vi "Error Query.vi"(8 "error in (no error)":errorcluster, 10 "Instrument Message":string[](array[string]), 11 "VISA resource name":refnum<visa-resource-name>) -> (0 "error out":errorcluster, 1 "Error Message":string, 2 "Error Code":i32[](array[numeric]), 3 "VISA resource out":refnum<visa-resource-name>)   [LabVIEW 2011, in "Hokuyo URG Series.lvlib"]
doc: "This VI checks the echo and status byte returned by URG commands and returns an error if one has occured. This VI is only called within the query instrument VI. The error codes used by this driver are documented on the Block Diagram of this VI."
uses:
  Hokuyo URG Series.lvlib
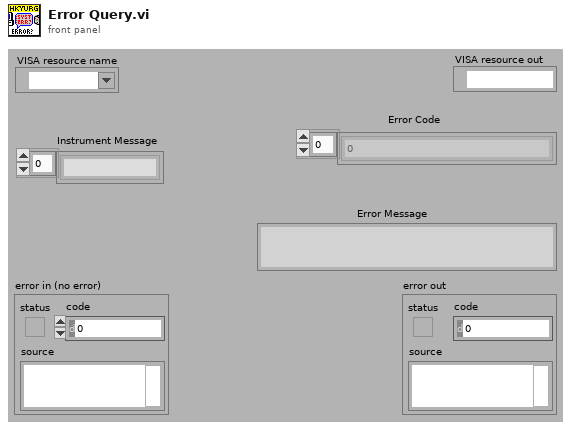
[diagram p1: front panel]
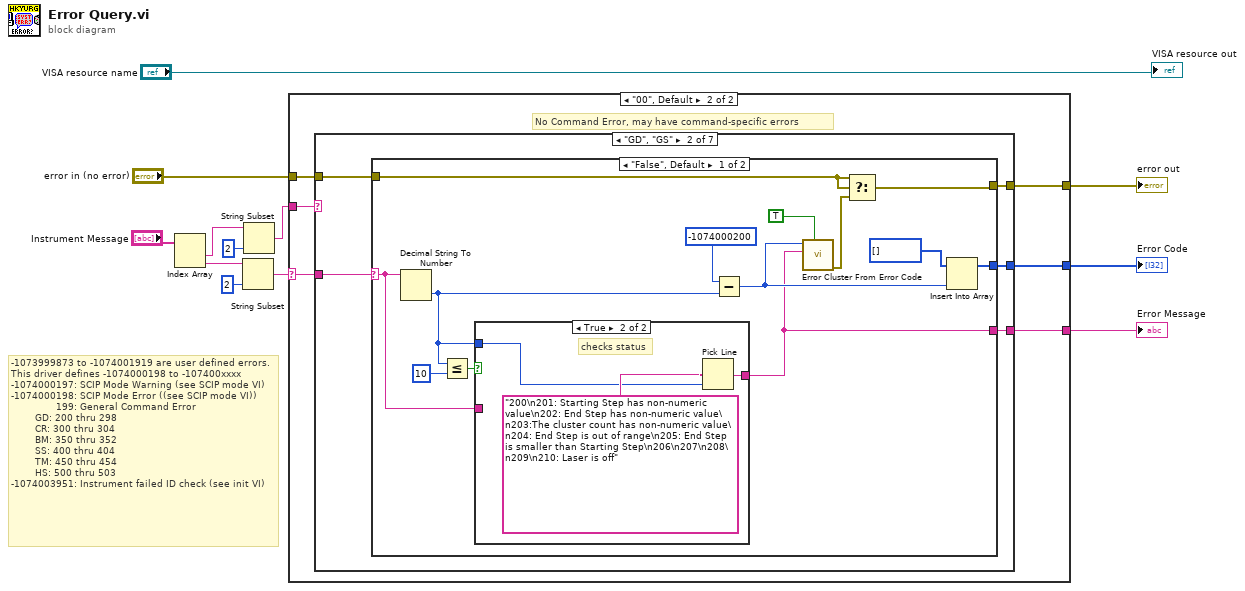
[diagram p0: block diagram]
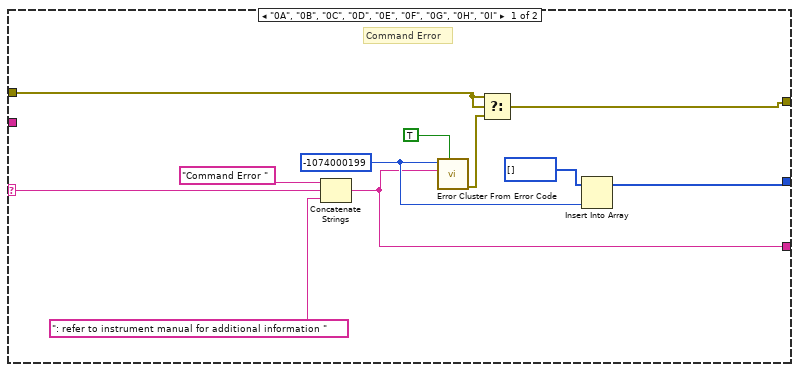
[diagram p2: hidden frame]
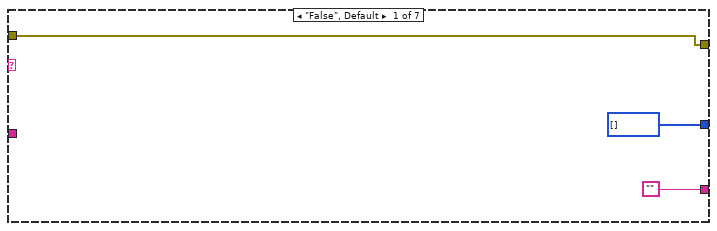
[diagram p3: hidden frame]
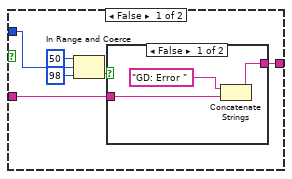
[diagram p4: hidden frame]
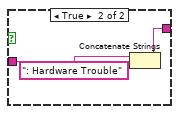
[diagram p5: hidden frame]
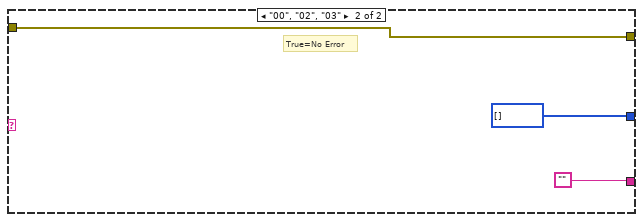
[diagram p6: hidden frame]
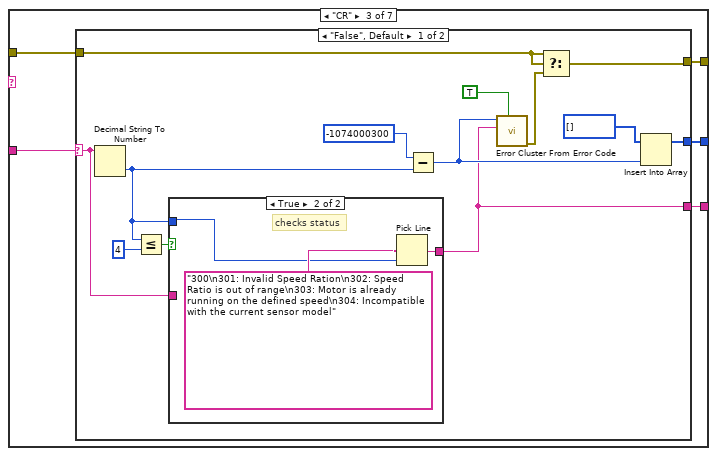
[diagram p7: hidden frame]
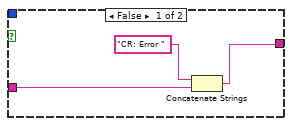
[diagram p8: hidden frame]
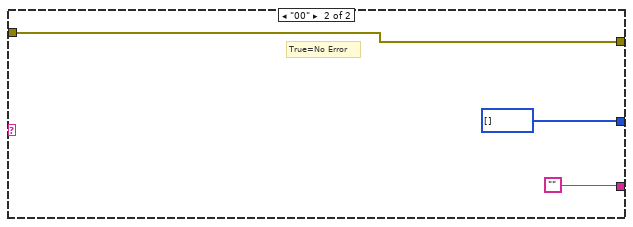
[diagram p9: hidden frame]
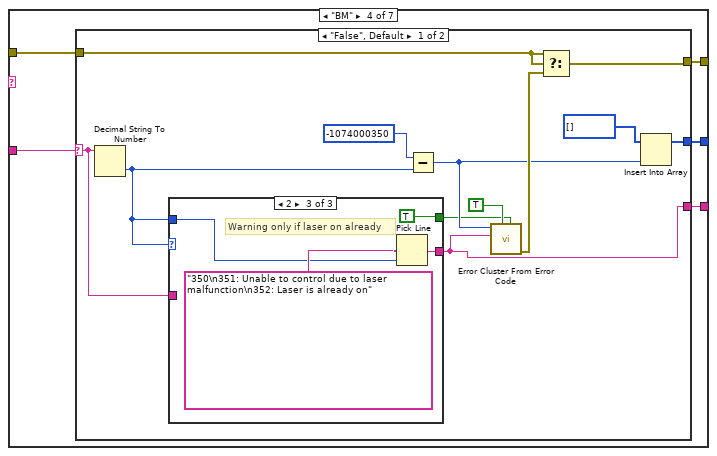
[diagram p10: hidden frame]
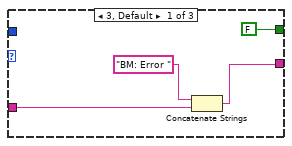
[diagram p11: hidden frame]
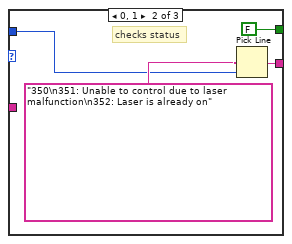
[diagram p12: hidden frame]
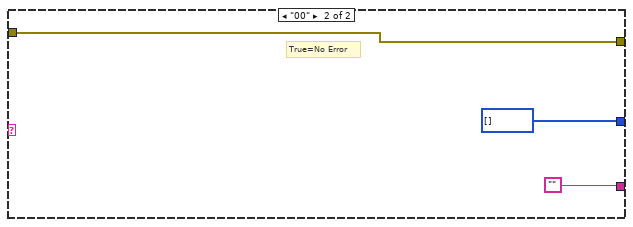
[diagram p13: hidden frame]
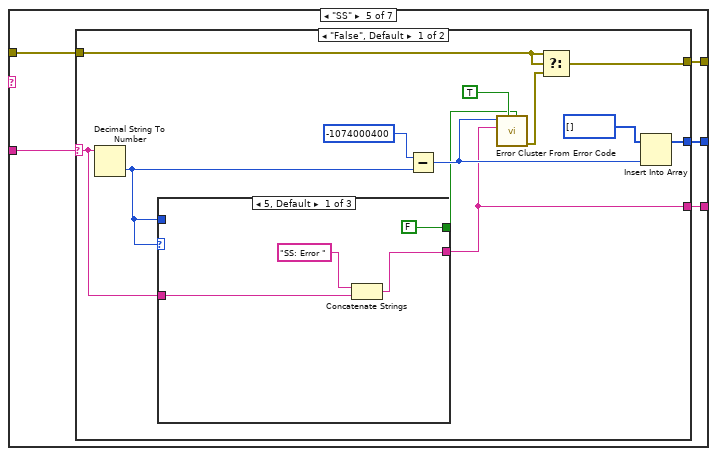
[diagram p14: hidden frame]
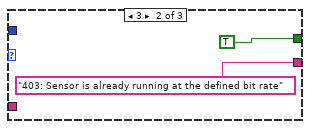
[diagram p15: hidden frame]
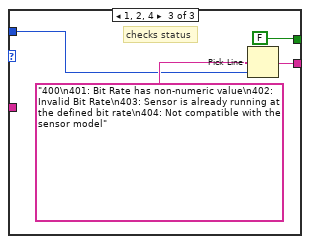
[diagram p16: hidden frame]
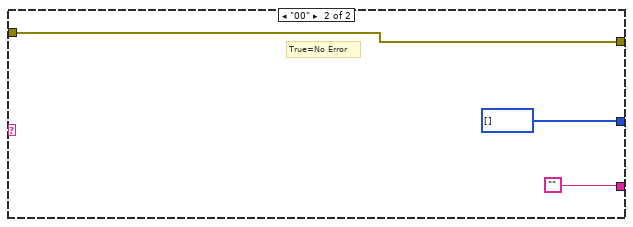
[diagram p17: hidden frame]
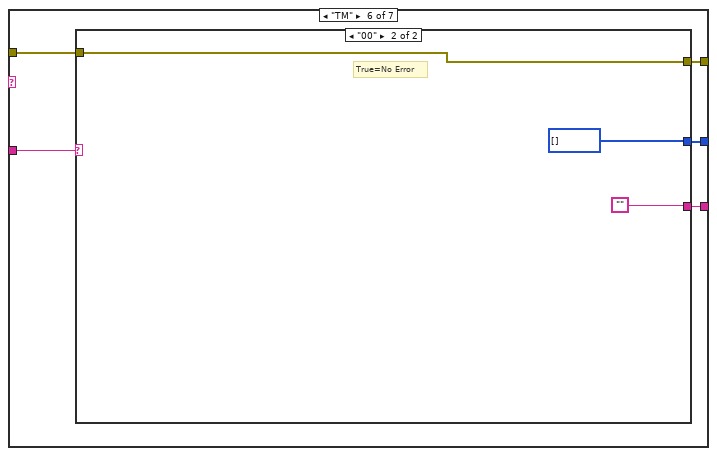
[diagram p18: hidden frame]
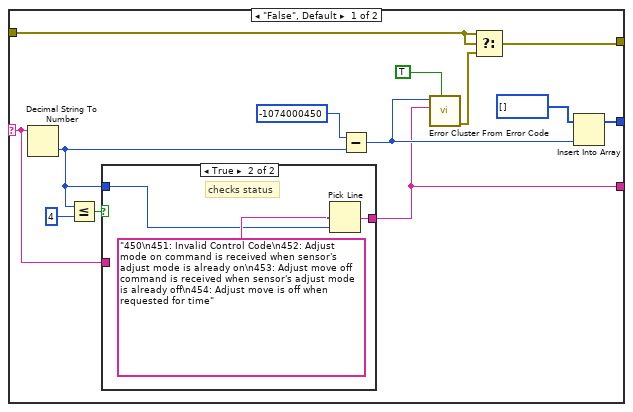
[diagram p19: hidden frame]
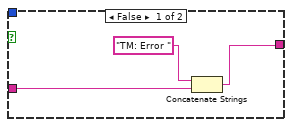
[diagram p20: hidden frame]
diagram:
  # "-1073999873 to -1074001919 are user defined errors.  This driver defines -1074000198 to -107400xxxx\n-1074000197: SCIP Mode Warning (see SCIP mode VI)\n-1074000198: SCIP Mode Error ((see SCIP mode VI))\n               199: General Command Error\n        GD: 200 thru 298\n        CR: 300 thru 304\n        BM: 350 thru 352\n        SS: 400 thru 404\n        TM: 450 thru 454\n        HS: 500 thru 503\n-1074003951: Instrument failed ID check (see init VI)"
  n1 = Index Array(array="Instrument Message") -> (element #1=w3:string, element #2=w4:string)  [unwired: 2 in]
  n2 = String Subset(string=w4, length (rest)=2 ("length (rest)")) -> (substring=w5:string)  [unwired: 1 in]
  n3 = String Subset(string=w3, length (rest)=2 ("length (rest)")) -> (substring=w1:string)  [unwired: 1 in]
  n4 = case shown="\"00\", Default" w5 {
    selector: w5 -> [w16 w24]
    tunnel: [w20 w29] -> w12
    tunnel: [w17 w28] -> w11
    tunnel: [w14 w27] -> w10
    tunnel: "error in (no error)" -> [w19 w26]
    tunnel: w1 -> [_ w25]
    frame "0A", "0B", "0C", "0D", "0E", "0F", "0G", "0H", "0I" {
      w18 = -1074000199
      # "Command Error"
      n5 = Concatenate Strings("Command Error " ("error message (\"\")"), w16, ": refer to instrument manual for additional information " ("error message (\"\")")) -> (w14:string)
      n6 = call <vilib>:"Error Cluster From Error Code.vi"("show call chain? (False)"=TRUE, "error message (\"\")"=w14, "error code (0)"=w18) -> ("error out"=w22:errorcluster)  [unwired: 6 in]
      n7 = Select(t=w19, s=w19, f=w22) -> (s? t:f=w20:errorcluster)
      n8 = Insert Into Array(array=i32[] [], new element=w18) -> (w17:i32[])  [unwired: 1 in]
    }
    frame "00", Default {
      # "No Command Error, may have command-specific errors"
      n9 = case shown="\"GD\", \"GS\"" w25 {
        tunnel: [w32 w37 w73 w100 w132 w162 w189] -> w29
        tunnel: [i32[] [] w36 w72 w99 w131 w161 w188] -> w28
        tunnel: ["" w35 w71 w98 w130 w160 w187] -> w27
        tunnel: w26 -> [w32 w34 w70 w97 w129 w159 w186]
        tunnel: w24 -> [_ w33 w69 w96 w128 w158 w185]
        frame "False", Default {
        }
        frame "GD", "GS" {
          n10 = case shown="\"False\", Default" w33 {
            selector: w33 -> [w38 _]
            tunnel: w34 -> [w43 w66]
            tunnel: [w48 w66] -> w37
            tunnel: [w44 i32[] []] -> w36
            tunnel: [w40 ""] -> w35
            frame "False", Default {
              n11 = Decimal String To Number(string=w38) -> (number=w39:i32)  [unwired: 2 in, 1 out]
              n12 = Less Or Equal?(x=w39, y=10) -> (x <= y?=w41:bool)
              n13 = case shown="True" w41 {
                tunnel: [w52 w65] -> w40
                tunnel: w39 -> [w54 w63]
                tunnel: w38 -> [w51 _]
                frame False {
                  n14 = In Range and Coerce(upper limit=50, x=w54, lower limit=98) -> (In Range?=w53:bool)  [unwired: 1 out]
                  n15 = case shown="False" w53 {
                    tunnel: w51 -> [w59 w61]
                    tunnel: [w57 w62] -> w52
                    frame False {
                      n16 = Concatenate Strings("GD: Error " ("string"), w59) -> (w57:string)
                    }
                    frame True {
                      n17 = Concatenate Strings(w61, ": Hardware Trouble" ("string")) -> (w62:string)
                    }
                  }
                }
                frame True {
                  # "checks status"
                  n18 = Pick Line(multi-line string="200\n201: Starting Step has non-numeric value\n202: End Step has non-numeric value\n203:The cluster count has non-numeric value\n204: End Step is out of range\n205: End Step is smaller than Starting Step\n206\n207\n208\n209\n210: Laser is off" ("error message (\"\")"), line index=w63) -> (output string=w65:string)  [unwired: 1 in]
                }
              }
              n19 = Subtract(x=-1074000200, y=w39) -> (x-y=w45:i32)
              n20 = call <vilib>:"Error Cluster From Error Code.vi"("show call chain? (False)"=TRUE, "error message (\"\")"=w40, "error code (0)"=w45) -> ("error out"=w49:errorcluster)  [unwired: 6 in]
              n21 = Select(t=w43, s=w43, f=w49) -> (s? t:f=w48:errorcluster)
              n22 = Insert Into Array(array=i32[] [], new element=w45) -> (w44:i32[])  [unwired: 1 in]
            }
            frame "00", "02", "03" {
              # "True=No Error"
            }
          }
        }
        frame "CR" {
          n23 = case shown="\"False\", Default" w69 {
            selector: w69 -> [w75 _]
            tunnel: w70 -> [w79 w93]
            tunnel: [w84 w93] -> w73
            tunnel: [w80 i32[] []] -> w72
            tunnel: [w76 ""] -> w71
            frame "False", Default {
              n24 = Decimal String To Number(string=w75) -> (number=w74:i32)  [unwired: 2 in, 1 out]
              n25 = Less Or Equal?(x=w74, y=4) -> (x <= y?=w77:bool)
              n26 = case shown="True" w77 {
                tunnel: [w89 w92] -> w76
                tunnel: w75 -> [w87 _]
                tunnel: w74 -> [_ w90]
                frame False {
                  n27 = Concatenate Strings("CR: Error " ("string"), w87) -> (w89:string)
                }
                frame True {
                  # "checks status"
                  n28 = Pick Line(multi-line string="300\n301: Invalid Speed Ration\n302: Speed Ratio is out of range\n303: Motor is already running on the defined speed\n304: Incompatible with the current sensor model" ("error message (\"\")"), line index=w90) -> (output string=w92:string)  [unwired: 1 in]
                }
              }
              n29 = Subtract(x=-1074000300, y=w74) -> (x-y=w81:i32)
              n30 = call <vilib>:"Error Cluster From Error Code.vi"("show call chain? (False)"=TRUE, "error message (\"\")"=w76, "error code (0)"=w81) -> ("error out"=w85:errorcluster)  [unwired: 6 in]
              n31 = Select(t=w79, s=w79, f=w85) -> (s? t:f=w84:errorcluster)
              n32 = Insert Into Array(array=i32[] [], new element=w81) -> (w80:i32[])  [unwired: 1 in]
            }
            frame "00" {
              # "True=No Error"
            }
          }
        }
        frame "BM" {
          n33 = case shown="\"False\", Default" w96 {
            selector: w96 -> [w103 _]
            tunnel: w97 -> [w105 w125]
            tunnel: [w110 w125] -> w100
            tunnel: [w106 i32[] []] -> w99
            tunnel: [w104 ""] -> w98
            frame "False", Default {
              n34 = Decimal String To Number(string=w103) -> (number=w102:i32)  [unwired: 2 in, 1 out]
              n35 = case shown="2" w102 {
                tunnel: [w116 w120 w124] -> w104
                tunnel: w102 -> [_ w118 w122]
                tunnel: w103 -> [w114 _ _]
                tunnel: [FALSE ("show call chain? (False)") FALSE ("show call chain? (False)") TRUE ("show call chain? (False)")] -> w101
                frame 3, Default {
                  n36 = Concatenate Strings("BM: Error " ("string"), w114) -> (w116:string)
                }
                frame 0, 1 {
                  # "checks status"
                  n37 = Pick Line(multi-line string="350\n351: Unable to control due to laser malfunction\n352: Laser is already on" ("error message (\"\")"), line index=w118) -> (output string=w120:string)  [unwired: 1 in]
                }
                frame 2 {
                  # "Warning only if laser on already"
                  n38 = Pick Line(multi-line string="350\n351: Unable to control due to laser malfunction\n352: Laser is already on" ("error message (\"\")"), line index=w122) -> (output string=w124:string)  [unwired: 1 in]
                }
              }
              n39 = Subtract(x=-1074000350, y=w102) -> (x-y=w107:i32)
              n40 = call <vilib>:"Error Cluster From Error Code.vi"("is warning? (False)"=w101, "show call chain? (False)"=TRUE, "error message (\"\")"=w104, "error code (0)"=w107) -> ("error out"=w111:errorcluster)  [unwired: 5 in]
              n41 = Select(t=w105, s=w105, f=w111) -> (s? t:f=w110:errorcluster)
              n42 = Insert Into Array(array=i32[] [], new element=w107) -> (w106:i32[])  [unwired: 1 in]
            }
            frame "00" {
              # "True=No Error"
            }
          }
        }
        frame "SS" {
          n43 = case shown="\"False\", Default" w128 {
            selector: w128 -> [w135 _]
            tunnel: w129 -> [w137 w155]
            tunnel: [w142 w155] -> w132
            tunnel: [w138 i32[] []] -> w131
            tunnel: [w136 ""] -> w130
            frame "False", Default {
              n44 = Decimal String To Number(string=w135) -> (number=w134:i32)  [unwired: 2 in, 1 out]
              n45 = case shown="5, Default" w134 {
                tunnel: [w148 "403: Sensor is already running at the defined bit rate" ("output string") w154] -> w136
                tunnel: w134 -> [_ _ w152]
                tunnel: w135 -> [w146 _ _]
                tunnel: [FALSE ("show call chain? (False)") TRUE ("show call chain? (False)") FALSE ("show call chain? (False)")] -> w133
                frame 5, Default {
                  n46 = Concatenate Strings("SS: Error " ("string"), w146) -> (w148:string)
                }
                frame 3 {
                }
                frame 1, 2, 4 {
                  # "checks status"
                  n47 = Pick Line(multi-line string="400\n401: Bit Rate has non-numeric value\n402: Invalid Bit Rate\n403: Sensor is already running at the defined bit rate\n404: Not compatible with the sensor model" ("error message (\"\")"), line index=w152) -> (output string=w154:string)  [unwired: 1 in]
                }
              }
              n48 = Subtract(x=-1074000400, y=w134) -> (x-y=w139:i32)
              n49 = call <vilib>:"Error Cluster From Error Code.vi"("is warning? (False)"=w133, "show call chain? (False)"=TRUE, "error message (\"\")"=w136, "error code (0)"=w139) -> ("error out"=w143:errorcluster)  [unwired: 5 in]
              n50 = Select(t=w137, s=w137, f=w143) -> (s? t:f=w142:errorcluster)
              n51 = Insert Into Array(array=i32[] [], new element=w139) -> (w138:i32[])  [unwired: 1 in]
            }
            frame "00" {
              # "True=No Error"
            }
          }
        }
        frame "TM" {
          n52 = case shown="\"00\"" w158 {
            selector: w158 -> [w163 _]
            tunnel: w159 -> [w168 w182]
            tunnel: [w173 w182] -> w162
            tunnel: [w169 i32[] []] -> w161
            tunnel: [w165 ""] -> w160
            frame "False", Default {
              n53 = Decimal String To Number(string=w163) -> (number=w164:i32)  [unwired: 2 in, 1 out]
              n54 = Less Or Equal?(x=w164, y=4) -> (x <= y?=w166:bool)
              n55 = case shown="True" w166 {
                tunnel: [w178 w181] -> w165
                tunnel: w164 -> [_ w179]
                tunnel: w163 -> [w176 _]
                frame False {
                  n56 = Concatenate Strings("TM: Error " ("string"), w176) -> (w178:string)
                }
                frame True {
                  # "checks status"
                  n57 = Pick Line(multi-line string="450\n451: Invalid Control Code\n452: Adjust mode on command is received when sensor's adjust mode is already on\n453: Adjust move off command is received when sensor's adjust mode is already off\n454: Adjust move is off when requested for time" ("error message (\"\")"), line index=w179) -> (output string=w181:string)  [unwired: 1 in]
                }
              }
              n58 = Subtract(x=-1074000450, y=w164) -> (x-y=w170:i32)
              n59 = call <vilib>:"Error Cluster From Error Code.vi"("show call chain? (False)"=TRUE, "error message (\"\")"=w165, "error code (0)"=w170) -> ("error out"=w174:errorcluster)  [unwired: 6 in]
              n60 = Select(t=w168, s=w168, f=w174) -> (s? t:f=w173:errorcluster)
              n61 = Insert Into Array(array=i32[] [], new element=w170) -> (w169:i32[])  [unwired: 1 in]
            }
            frame "00" {
              # "True=No Error"
            }
          }
        }
        frame "HS" {
          n62 = case shown="\"False\", Default" w185 {
            selector: w185 -> [w192 _]
            tunnel: w186 -> [w194 w214]
            tunnel: [w199 w214] -> w189
            tunnel: [w195 i32[] []] -> w188
            tunnel: [w193 ""] -> w187
            frame "False", Default {
              n63 = Decimal String To Number(string=w192) -> (number=w191:i32)  [unwired: 2 in, 1 out]
              n64 = case shown="0, 1, 3" w191 {
                tunnel: [w205 w209 w213] -> w193
                tunnel: w191 -> [_ w207 w211]
                tunnel: w192 -> [w203 _ _]
                tunnel: [FALSE ("show call chain? (False)") FALSE ("show call chain? (False)") TRUE ("show call chain? (False)")] -> w190
                frame 4, Default {
                  n65 = Concatenate Strings("HS: Error " ("string"), w203) -> (w205:string)
                }
                frame 0, 1, 3 {
                  # "checks status"
                  n66 = Pick Line(multi-line string="500\n501: Parameter Error\n502: Already running on the set mode\n503: Incompatible with current sensor model" ("error message (\"\")"), line index=w207) -> (output string=w209:string)  [unwired: 1 in]
                }
                frame 2 {
                  # "Warning only if already\nin set mode"
                  n67 = Pick Line(multi-line string="500\n501: Parameter Error\n502: Already running on the set mode\n503: Incompatible with current sensor model" ("error message (\"\")"), line index=w211) -> (output string=w213:string)  [unwired: 1 in]
                }
              }
              n68 = Subtract(x=-1074000500, y=w191) -> (x-y=w196:i32)
              n69 = call <vilib>:"Error Cluster From Error Code.vi"("is warning? (False)"=w190, "show call chain? (False)"=TRUE, "error message (\"\")"=w193, "error code (0)"=w196) -> ("error out"=w200:errorcluster)  [unwired: 5 in]
              n70 = Select(t=w194, s=w194, f=w200) -> (s? t:f=w199:errorcluster)
              n71 = Insert Into Array(array=i32[] [], new element=w196) -> (w195:i32[])  [unwired: 1 in]
            }
            frame "00" {
              # "True=No Error"
            }
          }
        }
      }
    }
  }
  "error out" <- w12
  "Error Code" <- w11
  "Error Message" <- w10
  "VISA resource out" <- "VISA resource name"
